vi "Time.vi"(8 "error in (no error)":errorcluster, 10 "Control In":T1={"I-O.lvclass"=refnum, "Gantry"=refnum, "Dispenser"="COM1"}, 11 "C4 Dispense in":refnum<class "Iterative Dispense.lvclass">) -> (0 "error out":errorcluster, 1 "Timing Data":i32[](array[numeric]), 2 "Control Out":T1={"I-O.lvclass"=refnum, "Gantry"=refnum, "Dispenser"="COM1"}, 3 "C4 Dispense out":refnum<class "Iterative Dispense.lvclass">)   [LabVIEW 2018, in "Iterative Dispense.lvclass"]
uses:
  Iterative Dispense.lvclass
  C:/Users/HEP/Documents/GitHub/New folder/C/Users/HEP/Documents/GitHub/UCSB-Gantry-HEP-2018/Classes/Routine/Dispense/Dispense.lvclass
  Controller/Controllers.ctl
  Controller/I-O/I-O.lvclass
  C:/Program Files (x86)/Aerotech/A3200/LabVIEW/2010/Bin/Aerotech.A3200.dll
  Program Files (x86)/Aerotech/A3200/LabVIEW/2010/Bin/Aerotech.A3200.dll
  Iterative Dispense.lvclass/Iterative Dispense.ctl
  Controller/Motion/Motion.lvclass
  Controller/Motion/A3200/A3200.lvclass
  Controller/Controller.lvclass
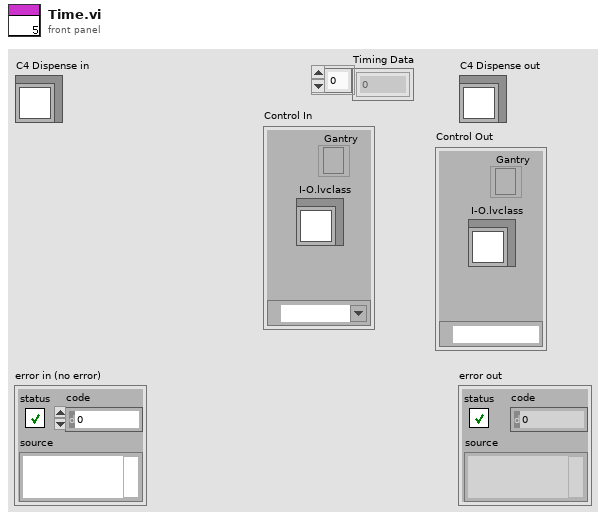
[diagram p1: front panel]
types:
  T1 = typedef "Controller.lvclass/Controllers.ctl" = cluster{"I-O.lvclass":refnum<class "I-O.lvclass">, "Gantry":refnum<k24>, "Dispenser":refnum<visa-resource-name>}
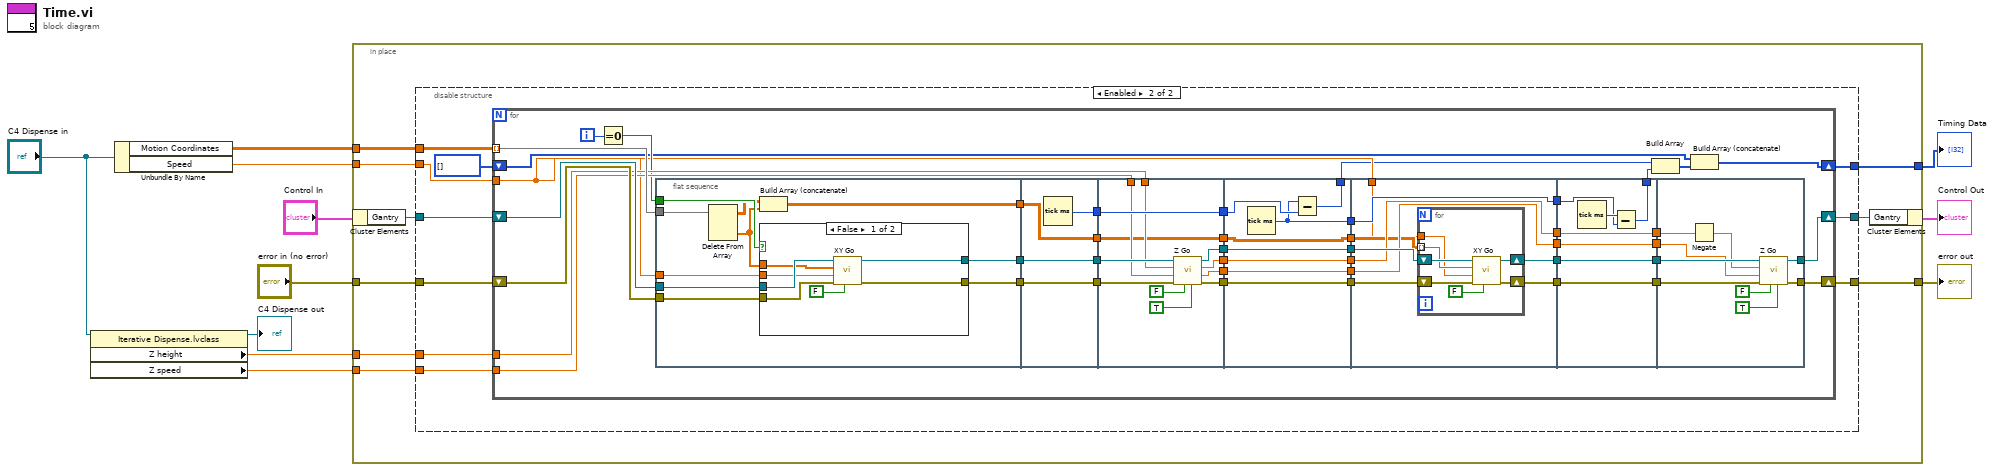
[diagram p0: block diagram]
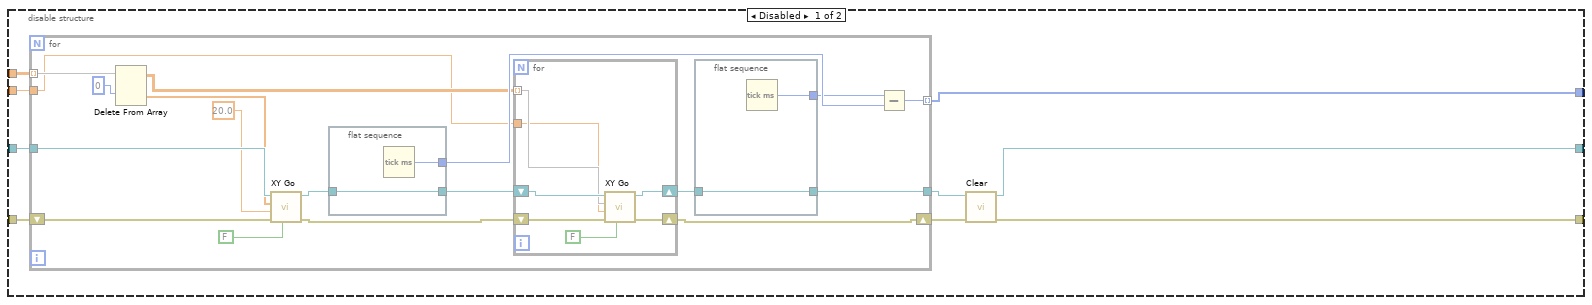
[diagram p2: hidden frame]
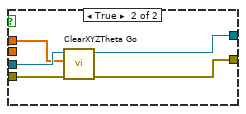
[diagram p3: hidden frame]
diagram:
  n1 = property class="Iterative Dispense.lvclass"(reference="C4 Dispense in") -> (reference out=→"C4 Dispense out":refnum<class "Iterative Dispense.lvclass">, "Z height"=w1:dbl, "Z speed"=w2:dbl)  [unwired: 1 in, 1 out]
  n2 = Unbundle By Name("C4 Dispense in") -> ("Motion Coordinates"=w11:dbl[][][], "Speed"=w7:dbl)
  n3 = in-place {
    in-place-border: w11 -> [w20]
    in-place-border: [w19] -> w10
    in-place-border: w7 -> [w18]
    in-place-border: "error in (no error)" -> [w15]
    in-place-border: [w14] -> w5
    in-place-border: w2 -> [w13]
    in-place-border: w1 -> [w12]
    n4 = in-place-cluster #1("Control In") -> ("Gantry"=w17:refnum<k24>)
    n5 = disable-structure shown="Enabled" {
      disable-tunnel: w20 -> [w29 w68]
      disable-tunnel: [w28 w60] -> w19
      disable-tunnel: w18 -> [w27 w63]
      disable-tunnel: w17 -> [w26 w67]
      disable-tunnel: [w25 w62] -> w16
      disable-tunnel: w15 -> [w23 w66]
      disable-tunnel: [w21 w61] -> w14
      disable-tunnel: w13 -> [_ w65]
      disable-tunnel: w12 -> [_ w64]
      frame Disabled {
        n6 = for {
          tunnel: [w45] -> w28 mode=indexing
          tunnel: w29 -> [w42] mode=indexing
          tunnel: w27 -> [w41]
          tunnel: w26 -> [w39]
          tunnel: [w36] -> w24
          shift-right: [w31] -> w22
          shift-left: w23 -> [w33]
          n7 = Delete From Array(array=w42, index (row)=0) -> (deleted portion=w35:dbl[], array with subset deleted=w44:dbl[][])  [unwired: 2 in]
          n8 = call "XY Go.vi"("return immediately"=FALSE, "error in (no error)"=w33, "Speed"=20.0, "XY In"=w35, "Gantry In"=w39) -> ("error out"=w32:errorcluster, "Gantry Out"=w38:refnum<k24>)  [unwired: 4 in, 1 out]
          n9 = flat-sequence {
            tunnel: [w51] -> w47
            tunnel: w38 -> [w50]
            tunnel: [w50] -> w37
            frame #0 {
              n10 = Tick Count (ms)() -> (millisecond timer value=w51:u32)
            }
          }
          n11 = for {
            tunnel: w44 -> [w56] mode=indexing
            tunnel: w41 -> [w55]
            shift-right: [w57] -> w40
            shift-left: w37 -> [w58]
            shift-right: [w53] -> w31
            shift-left: w32 -> [w54]
            n12 = call "XY Go.vi"("return immediately"=FALSE, "error in (no error)"=w54, "Speed"=w55, "XY In"=w56, "Gantry In"=w58) -> ("error out"=w53:errorcluster, "Gantry Out"=w57:refnum<k24>)  [unwired: 4 in, 1 out]
          }
          n13 = flat-sequence {
            tunnel: [w49] -> w46
            tunnel: [w48] -> w36
            tunnel: w40 -> [w48]
            frame #0 {
              n14 = Tick Count (ms)() -> (millisecond timer value=w49:u32)
            }
          }
          n15 = Subtract(x=w46, y=w47) -> (x-y=w45:u32)
        }
        n16 = call "Clear.vi"("error in (no error)"=w22, "Gantry In"=w24) -> ("error out"=w21:errorcluster, "Gantry Out"=w25:refnum<k24>)  [unwired: 8 in]
      }
      frame Enabled {
        n17 = for {
          tunnel: w68 -> [w86] mode=indexing
          tunnel: w65 -> [w84]
          tunnel: w64 -> [w83]
          tunnel: w63 -> [w74]
          shift-right: [w78] -> w62
          shift-left: w67 -> [w87]
          shift-right: [w77] -> w61
          shift-left: w66 -> [w85]
          shift-right: [w69] -> w60
          shift-left: u32[] [] -> [w72]
          i -> [w76]
          n18 = Equal To 0?(x=w76) -> (x = 0?=w75:bool)
          n19 = flat-sequence {
            tunnel: [w121] -> w111
            tunnel: [w120] -> w110
            tunnel: w87 -> [w119]
            tunnel: w86 -> [w118]
            tunnel: w85 -> [w117]
            tunnel: [w112] -> w79
            tunnel: w75 -> [w116]
            tunnel: w74 -> [w115]
            tunnel: w111 -> [w136]
            tunnel: [w136] -> w109
            tunnel: [w137] -> w108
            tunnel: [w135] -> w107
            tunnel: w110 -> [w135]
            tunnel: [w134] -> w80
            tunnel: w79 -> [w134]
            tunnel: w109 -> [w149]
            tunnel: [w148] -> w106
            tunnel: w108 -> [w148]
            tunnel: [w147] -> w105
            tunnel: [w146] -> w104
            tunnel: [w145] -> w103
            tunnel: w107 -> [w144]
            tunnel: [w143] -> w102
            tunnel: w84 -> [w140]
            tunnel: w83 -> [w139]
            tunnel: [w138] -> w81
            tunnel: w80 -> [w138]
            tunnel: w106 -> [w157]
            tunnel: [w156] -> w70
            tunnel: [w155] -> w101
            tunnel: w105 -> [w155]
            tunnel: [w154] -> w100
            tunnel: [w153] -> w99
            tunnel: w104 -> [w153]
            tunnel: [w152] -> w98
            tunnel: w103 -> [w152]
            tunnel: w102 -> [w151]
            tunnel: [w151] -> w97
            tunnel: [w150] -> w82
            tunnel: w81 -> [w150]
            tunnel: w101 -> [w166]
            tunnel: [w165] -> w96
            tunnel: w100 -> [w165]
            tunnel: [w164] -> w95
            tunnel: [w163] -> w94
            tunnel: w99 -> [w163]
            tunnel: [w162] -> w93
            tunnel: w98 -> [w162]
            tunnel: w97 -> [w161]
            tunnel: [w160] -> w92
            tunnel: w82 -> [w159]
            tunnel: w74 -> [w158]
            tunnel: w96 -> [w179]
            tunnel: [w178] -> w91
            tunnel: w95 -> [w178]
            tunnel: [w177] -> w90
            tunnel: w94 -> [w177]
            tunnel: [w176] -> w89
            tunnel: w93 -> [w176]
            tunnel: [w175] -> w88
            tunnel: w92 -> [w175]
            tunnel: [w174] -> w71
            tunnel: w91 -> [w189]
            tunnel: w90 -> [w188]
            tunnel: w89 -> [w186]
            tunnel: [w185] -> w78
            tunnel: w88 -> [w184]
            tunnel: [w183] -> w77
            frame #0 {
              n20 = Delete From Array(array=w118) -> (deleted portion=w113:dbl[], array with subset deleted=w114:dbl[][])  [unwired: 3 in]
              n21 = Build Array (concatenate)(w114, w113) -> (w112:dbl[][])
              n22 = case shown="False" w116 {
                tunnel: [w128 w133] -> w121
                tunnel: [w127 w132] -> w120
                tunnel: w119 -> [w124 w131]
                tunnel: w113 -> [w123 w130]
                tunnel: w117 -> [w125 w129]
                tunnel: w115 -> [w122 _]
                frame False {
                  n23 = call "XY Go.vi"("return immediately"=FALSE, "error in (no error)"=w125, "Speed"=w122, "XY In"=w123, "Gantry In"=w124) -> ("error out"=w127:errorcluster, "Gantry Out"=w128:refnum<k24>)  [unwired: 4 in, 1 out]
                }
                frame True {
                  n24 = call "ClearXYZTheta Go.vi"("error in (no error)"=w129, "XYZTheta In"=w130, "Gantry In"=w131) -> ("error out"=w132:errorcluster, "Gantry Out"=w133:refnum<k24>)  [unwired: 6 in, 1 out]
                }
              }
            }
            frame #1 {
              n25 = Tick Count (ms)() -> (millisecond timer value=w137:u32)
            }
            frame #2 {
              n26 = call "Z Go.vi"("Increment"=TRUE, "Return Immediately"=FALSE, "error in (no error)"=w144, "Speed In"=w140, "Position In"=w139, "Gantry In"=w149) -> ("error out"=w143:errorcluster, "Speed Out"=w145:dbl, "Position Out"=w146:dbl, "Gantry Out"=w147:refnum<k24>)  [unwired: 2 in]
            }
            frame #3 {
              n27 = Tick Count (ms)() -> (millisecond timer value=w154:u32)
              n28 = Subtract(x=w154, y=w157) -> (x-y=w156:u32)
            }
            frame #4 {
              n29 = for {
                shift-right: [w172] -> w164
                shift-left: w166 -> [w173]
                shift-right: [w170] -> w160
                shift-left: w161 -> [w171]
                tunnel: w159 -> [w168] mode=indexing
                tunnel: w158 -> [w167]
                n30 = call "XY Go.vi"("return immediately"=FALSE, "error in (no error)"=w171, "Speed"=w167, "XY In"=w168, "Gantry In"=w173) -> ("error out"=w170:errorcluster, "Gantry Out"=w172:refnum<k24>)  [unwired: 4 in, 1 out]
              }
            }
            frame #5 {
              n31 = Tick Count (ms)() -> (millisecond timer value=w180:u32)
              n32 = Subtract(x=w180, y=w179) -> (x-y=w174:u32)
            }
            frame #6 {
              n33 = Negate(x=w188) -> (-x=w187:dbl)
              n34 = call "Z Go.vi"("Increment"=TRUE, "Return Immediately"=FALSE, "error in (no error)"=w184, "Speed In"=w186, "Position In"=w187, "Gantry In"=w189) -> ("error out"=w183:errorcluster, "Gantry Out"=w185:refnum<k24>)  [unwired: 2 in, 2 out]
            }
          }
          n35 = Build Array(w70, w71) -> (w73:u32[])
          n36 = Build Array (concatenate)(w72, w73) -> (w69:u32[])
        }
      }
    }
    n37 = in-place-cluster #1("Gantry"=w16) -> (→"Control Out":T1)
  }
  "error out" <- w5
  "Timing Data" <- w10
